vi "Detect Line Change.vi"(9 "Original Tag":string, 10 "Original Line":T1 {"OPC UA Data Type" items=["Boolean"=1, "SByte"=2, "Byte"=3, "Int16"=4, "UInt16"=5, "Int32"=6, "UInt32"=7, "Int64"=8, "UInt64"=9, "Float"=10, "Double"=11, "String"=12, "DateTime"=13, "ByteString"=15, "Array of Boolean"=101, "Array of SByte"=102, "Array of Byte"=103, "Array of Int16"=104, "Array of UInt16"=105, "Array of Int32"=106, "Array of UInt32"=107, "Array of Int64"=108, "Array of UInt64"=109, "Array of Float"=110, "Array of Double"=111, "Array of String"=112, "Array of DateTime"=113, "Array of ByteString"=115]}, 11 "Mappings In":T3 {"Line"."OPC UA Data Type" items=["Boolean"=1, "SByte"=2, "Byte"=3, "Int16"=4, "UInt16"=5, "Int32"=6, "UInt32"=7, "Int64"=8, "UInt64"=9, "Float"=10, "Double"=11, "String"=12, "DateTime"=13, "ByteString"=15, "Array of Boolean"=101, "Array of SByte"=102, "Array of Byte"=103, "Array of Int16"=104, "Array of UInt16"=105, "Array of Int32"=106, "Array of UInt32"=107, "Array of Int64"=108, "Array of UInt64"=109, "Array of Float"=110, "Array of Double"=111, "Array of String"=112, "Array of DateTime"=113, "Array of ByteString"=115]}) -> (2 "Changed?":bool, 3 "Mappings Out":T3 {"Line"."OPC UA Data Type" items=["Boolean"=1, "SByte"=2, "Byte"=3, "Int16"=4, "UInt16"=5, "Int32"=6, "UInt32"=7, "Int64"=8, "UInt64"=9, "Float"=10, "Double"=11, "String"=12, "DateTime"=13, "ByteString"=15, "Array of Boolean"=101, "Array of SByte"=102, "Array of Byte"=103, "Array of Int16"=104, "Array of UInt16"=105, "Array of Int32"=106, "Array of UInt32"=107, "Array of Int64"=108, "Array of UInt64"=109, "Array of Float"=110, "Array of Double"=111, "Array of String"=112, "Array of DateTime"=113, "Array of ByteString"=115]})   [LabVIEW 2014, in "OPC UA Client editor node.lvclass"]
doc: "Detect whether a change has occurred in the configure channel dialog window"
uses:
  OPC UA Client editor node.lvclass
  Mappings.ctl
  <vilib>/NI/Tag Bus Module Framework/channel/TBM channel.lvclass
  module/configuration/Line.ctl
  module/configuration/OPC UA Data Type.ctl
  Map.ctl
  module/configuration/OPC UA Client configuration.lvclass
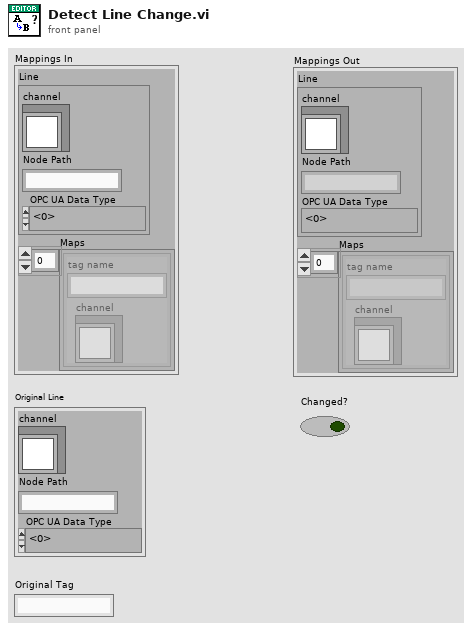
[diagram p1: front panel]
types:
  T1 = typedef "OPC UA Client configuration.lvclass/Line.ctl" = cluster{"channel":refnum<class "TBM channel.lvclass">, "Node Path":string, "OPC UA Data Type":T2}
  T2 = typedef "OPC UA Client configuration.lvclass/OPC UA Data Type.ctl" = u16
  T3 = typedef "OPC UA Client editor node.lvclass/Mappings.ctl" = cluster{"Line":T1, "Maps":T4[]}
  T4 = typedef "OPC UA Client editor node.lvclass/Map.ctl" = cluster{"channel":refnum<class "TBM channel.lvclass">, "tag name":string}
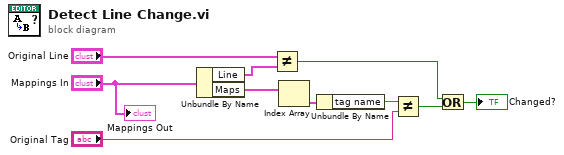
[diagram p0: block diagram]
diagram:
  n1 = Unbundle By Name("Mappings In") -> ("Line"=w9:T1, "Maps"=w7:T4[])
  n2 = Not Equal?(x="Original Line", y=w9) -> (x != y?=w2:bool)
  n3 = Index Array(array=w7) -> (element=w6:T4)  [unwired: 1 in]
  n4 = Unbundle By Name(w6) -> ("tag name"=w5:string)
  n5 = Not Equal?(x=w5, y="Original Tag") -> (x != y?=w3:bool)
  n6 = Or(x=w2, y=w3) -> (x .or. y?=→"Changed?":bool)
  "Mappings Out" <- "Mappings In"
